vi "S2C_ExeScriptPreAbort.vi"(8 "Error In":errorcluster, 11 "Q-Ref":refnum<queue>) -> (0 "Error Out":errorcluster)   [LabVIEW 2015]
uses:
  Globals/S2C_Globals.vi
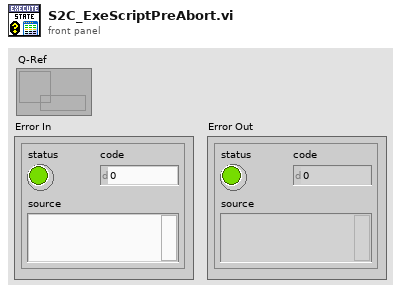
[diagram p1: front panel]
types:
  T1 = enum8{"Enabled", "Disabled", "Disabled and Grayed Out"}
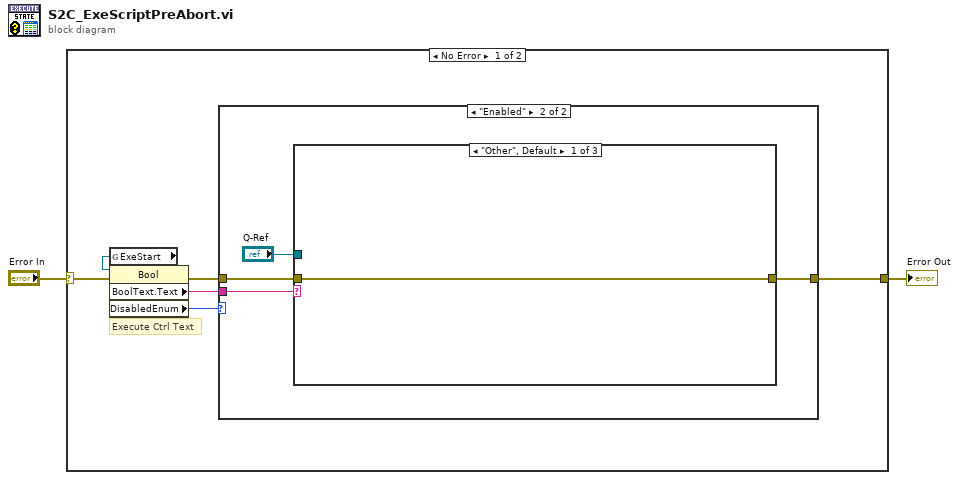
[diagram p0: block diagram]
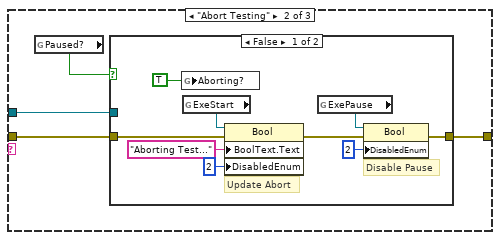
[diagram p3: hidden frame]
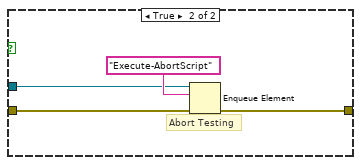
[diagram p4: hidden frame]
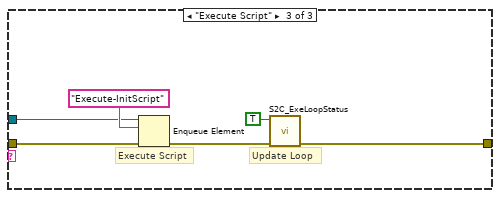
[diagram p5: hidden frame]
diagram:
  n1 = case shown="No Error" "Error In" {
    selector: "Error In" -> [w7 w37]
    tunnel: [w4 w37] -> w1
    frame No Error {
      # "Execute Ctrl Text"
      n2 = global read "S2C_Globals.vi" "ExeStart"() -> (w6:refnum<vi>)
      n3 = property on="Property Node" class="Bool"(reference=w6) -> ("BoolText.Text"=w5:string, "DisabledEnum"=w3:T1)  [unwired: 1 in, 2 out]
      n4 = case shown="\"Enabled\"" w3 {
        tunnel: w7 -> [w8 w12]
        tunnel: w5 -> [_ w11]
        tunnel: [w8 w9] -> w4
        frame "Disabled", Default {
        }
        frame "Enabled" {
          n5 = case shown="\"Other\", Default" w11 {
            tunnel: w12 -> [w13 w17 w35]
            tunnel: "Q-Ref" -> [_ w14 w34]
            tunnel: [w13 w16 w31] -> w9
            frame "Other", Default {
            }
            frame "Abort Testing" {
              n6 = global read "S2C_Globals.vi" "Paused?"() -> (w15:bool)
              n7 = case shown="False" w15 {
                tunnel: w17 -> [w21 w29]
                tunnel: [w19 w27] -> w16
                tunnel: w14 -> [_ w28]
                frame False {
                  # "Update Abort"
                  # "Disable Pause"
                  n8 = global write "S2C_Globals.vi" "Aborting?"(TRUE ("Aborting?")) -> ()
                  n9 = global read "S2C_Globals.vi" "ExeStart"() -> (w24:refnum<vi>)
                  n10 = property on="Property Node" class="Bool"(reference=w24, error in=w21, "BoolText.Text"="Aborting Test..." ("Boolean Text.Text"), "DisabledEnum"=u8 2) -> (error out=w22:errorcluster)  [unwired: 1 out]
                  n11 = global read "S2C_Globals.vi" "ExePause"() -> (w26:refnum<vi>)
                  n12 = property on="Property Node" class="Bool"(reference=w26, error in=w22, "DisabledEnum"=u8 2) -> (error out=w19:errorcluster)  [unwired: 1 out]
                }
                frame True {
                  # "Abort Testing"
                  n13 = Enqueue Element(queue=w28, element="Execute-AbortScript", error in (no error)=w29) -> (error out=w27:errorcluster)  [unwired: 1 in, 2 out]
                }
              }
            }
            frame "Execute Script" {
              # "Update Loop"
              # "Execute Script"
              n14 = Enqueue Element(queue=w34, element="Execute-InitScript", error in (no error)=w35) -> (error out=w32:errorcluster)  [unwired: 1 in, 2 out]
              n15 = call "S2C_ExeLoopStatus.vi"("Error In"=w32, "Reset?"=TRUE) -> ("Error Out"=w31:errorcluster)  [unwired: 9 in]
            }
          }
        }
      }
    }
    frame Error {
    }
  }
  "Error Out" <- w1
